vi "MeanofTIFF.vi"(11 "file path":path) -> (0 "read error":errorcluster)   [LabVIEW 2011]
uses:
  tiff/TiffModules/ReadTiffPage_I16_text.vi
panel:
  out "Write error":errorcluster
  out "Numeric":i32
  # "Mean of all planes\nOutput will be Name_Mean.tif"
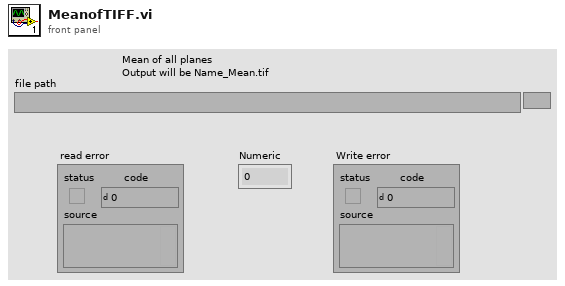
[diagram p1: front panel]
types:
  T1 = cluster{"Tiff refnum":refnum<file>, "BigTiff,Endian":u16}
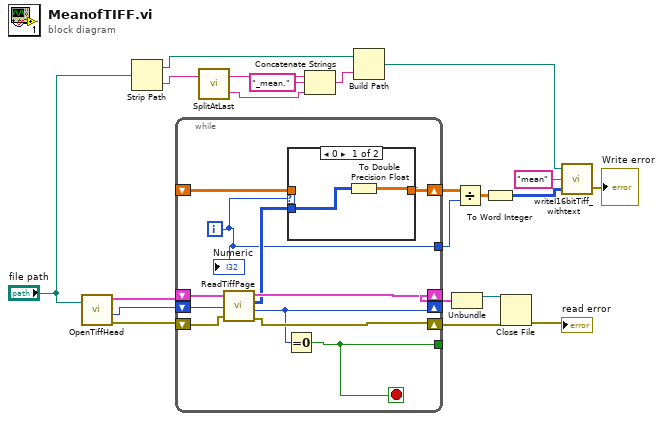
[diagram p0: block diagram]
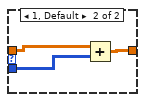
[diagram p2: hidden frame]
diagram:
  n1 = call "OpenTiffHead.vi"("file path"="file path") -> ("TIFF file"=w20:T1, "first Diroffset"=w21:u64, "error out"=w19:errorcluster)  [unwired: 2 in]
  n2 = Strip Path(path="file path") -> (stripped path=w9:path, name=w13:string)
  n3 = while {
    shift-right: [w26] -> _
    shift-left: w21 -> [w32]
    shift-right: [w28] -> w16
    shift-left: w20 -> [w31]
    shift-right: [w29] -> w15
    shift-left: w19 -> [w30]
    tunnel: [w27] -> _
    shift-right: [w24] -> w7
    shift-left: _ -> [w23]
    tunnel: [w22] -> w6
    i -> [w22]
    stop <- w27 stop-if-true
    n4 = call-poly "ReadTiffPage.vi"("TIFF file"=w31, "IFDoffset"=w32, "error in"=w30) -> ("TIFF file out"=w28:T1, "16-bit pixmap"=w25:i16[][], "Next offset"=w26:i64, "error out"=w29:errorcluster)  [unwired: 3 in, 1 out]
    n5 = Equal To 0?(x=w26) -> (x = 0?=w27:bool)
    n6 = case shown="0" w22 {
      tunnel: w25 -> [w34 w37]
      tunnel: [w33 w36] -> w24
      tunnel: w23 -> [_ w35]
      frame 0 {
        n7 = To Double Precision Float(number=w34) -> (double precision float=w33:dbl[][])
      }
      frame 1, Default {
        n8 = Add(x=w35, y=w37) -> (x+y=w36:dbl[][])
      }
    }
    "Numeric" <- w22
  }
  n9 = call "SplitAtLast.vi"("In-String"=w13) -> ("end"=w10:string, "Front (default)"=w12:string)  [unwired: 1 in]
  n10 = Concatenate Strings(w12, "_mean." ("string"), w10) -> (w8:string)
  n11 = Build Path(base path=w9, name or relative path=w8) -> (appended path=w4:path)
  n12 = Unbundle(w16) -> ("Tiff refnum"=w18:refnum<file>)  [unwired: 1 out]
  n13 = Divide(x=w7, y=w6) -> (x/y=w5:dbl[][])
  n14 = To Word Integer(number=w5) -> (16bit integer=w3:i16[][])
  n15 = Close File(refnum=w18, error in=w15) -> (error out=→"read error":errorcluster)  [unwired: 1 out]
  n16 = call "writeI16bitTiff_withtext.vi"("16-bit pixmap x, y"=w3, "Text"="mean", "file path"=w4) -> ("error out"=→"Write error":errorcluster)  [unwired: 1 in]
